vi "Car Model Types.vi"(0 "body":string) -> (1 "Car HTMLs":string[](array[string]), 2 "No of HTMLs":i32)   [LabVIEW 2018]
uses:
  <vilib>/httpClient/LabVIEWHTTPClient.lvlib
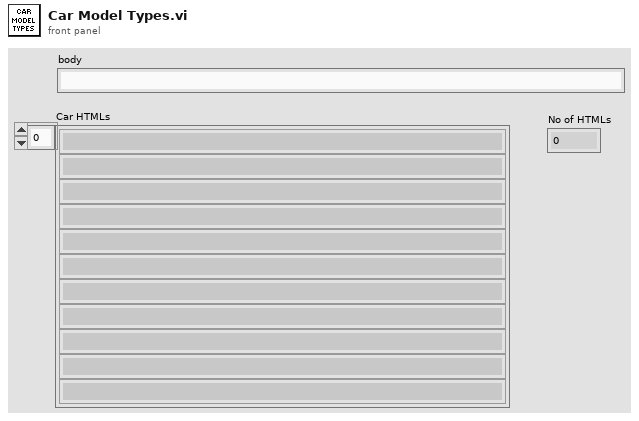
[diagram p1: front panel]
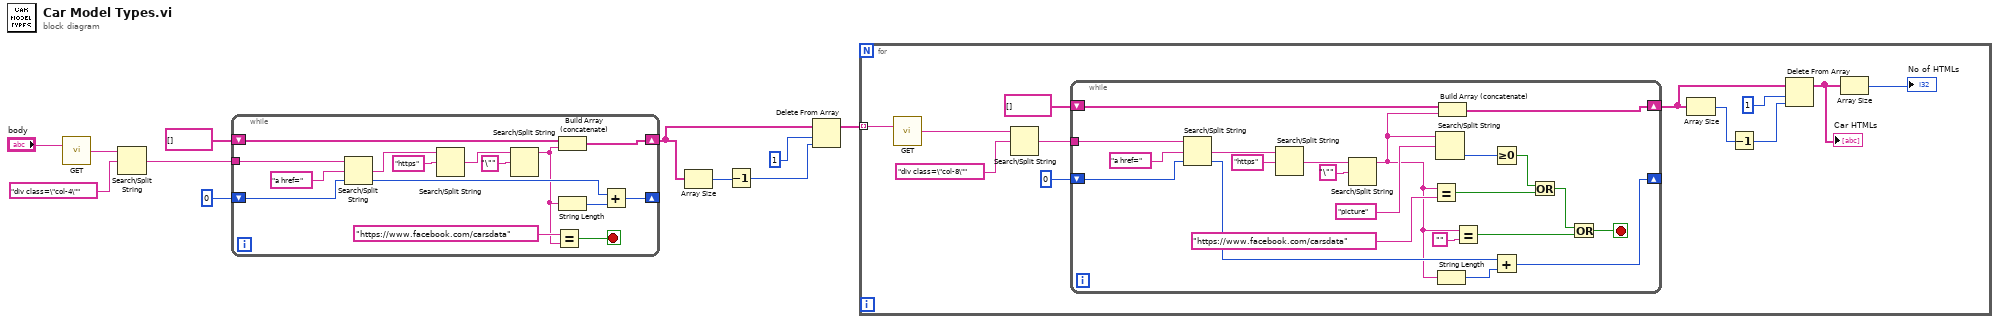
[diagram p0: block diagram]
diagram:
  n1 = call <vilib>:"GET.vi"("url"="body") -> ("body"=w8:string)  [unwired: 11 in, 3 out]
  n2 = Search/Split String(string=w8, search string/char (-)="div class=\"col-4\"") -> (match + rest of string=w11:string)  [unwired: 1 in, 2 out]
  n3 = while {
    tunnel: w11 -> [w24]
    shift-right: [w25] -> w2
    shift-left: string[] [] -> [w26]
    shift-right: [w17] -> _
    shift-left: 0 -> [w15]
    stop <- w14 stop-if-true
    n4 = Search/Split String(string=w24, search string/char (-)="a href=", offset (0)=w15) -> (match + rest of string=w19:string, offset of match=w16:i32)  [unwired: 1 out]
    n5 = Search/Split String(string=w19, search string/char (-)="https") -> (match + rest of string=w22:string)  [unwired: 1 in, 2 out]
    n6 = Search/Split String(string=w22, search string/char (-)="\"") -> (substring before match=w12:string)  [unwired: 1 in, 2 out]
    n7 = Equal?(x="https://www.facebook.com/carsdata", y=w12) -> (x = y?=w14:bool)
    n8 = Build Array (concatenate)(w26, w12) -> (w25:string[])
    n9 = String Length(string=w12) -> (length=w18:i32)
    n10 = Add(x=w16, y=w18) -> (x+y=w17:i32)
  }
  n11 = Array Size(array=w2) -> (size(s)=w4:i32)
  n12 = Decrement(x=w4) -> (x-1=w3:i32)
  n13 = Delete From Array(array=w2, length=1, index=w3) -> (array with subset deleted=w1:string[])  [unwired: 1 out]
  n14 = for {
    tunnel: w1 -> [w29] mode=indexing
    n15 = call <vilib>:"GET.vi"("url"=w29) -> ("body"=w35:string)  [unwired: 11 in, 3 out]
    n16 = Search/Split String(string=w35, search string/char (-)="div class=\"col-8\"") -> (match + rest of string=w38:string)  [unwired: 1 in, 2 out]
    n17 = while {
      tunnel: w38 -> [w58]
      shift-right: [w59] -> w30
      shift-left: string[] [] -> [w60]
      shift-right: [w51] -> _
      shift-left: 0 -> [w49]
      stop <- w39 stop-if-true
      n18 = Search/Split String(string=w58, search string/char (-)="a href=", offset (0)=w49) -> (match + rest of string=w53:string, offset of match=w50:i32)  [unwired: 1 out]
      n19 = Search/Split String(string=w53, search string/char (-)="https") -> (match + rest of string=w56:string)  [unwired: 1 in, 2 out]
      n20 = Search/Split String(string=w56, search string/char (-)="\"") -> (substring before match=w42:string)  [unwired: 1 in, 2 out]
      n21 = Equal?(x=w42, y="https://www.facebook.com/carsdata") -> (x = y?=w44:bool)
      n22 = Search/Split String(string=w42, search string/char (-)="picture") -> (offset of match=w47:i32)  [unwired: 1 in, 2 out]
      n23 = String Length(string=w42) -> (length=w52:i32)
      n24 = Build Array (concatenate)(w60, w42) -> (w59:string[])
      n25 = Equal?(x=w42, y="") -> (x = y?=w41:bool)
      n26 = Greater Or Equal To 0?(x=w47) -> (x >= 0?=w46:bool)
      n27 = Add(x=w50, y=w52) -> (x+y=w51:i32)
      n28 = Or(x=w46, y=w44) -> (x .or. y?=w40:bool)
      n29 = Or(x=w40, y=w41) -> (x .or. y?=w39:bool)
    }
    n30 = Array Size(array=w30) -> (size(s)=w32:i32)
    n31 = Decrement(x=w32) -> (x-1=w31:i32)
    n32 = Delete From Array(array=w30, length=1, index=w31) -> (array with subset deleted=w28:string[])  [unwired: 1 out]
    "Car HTMLs" <- w28
    n33 = Array Size(array=w28) -> (size(s)=→"No of HTMLs":i32)
  }
